vi "Main.vi"(8 "error in":errorcluster, 11 "DataBase in":refnum<class "DataBase.lvclass">) -> (0 "error out":errorcluster, 3 "DataBase out":refnum<class "DataBase.lvclass">)   [LabVIEW 2023, in "DataBase.lvclass"]
doc: "The <b>Queued Message Handler</b> of the Worker that owns this VI."
uses:
  DataBase.lvclass
  C:/Program Files/National Instruments/LabVIEW 2023/vi.lib/addons/_Workers/Library/Classes/Worker/Worker.lvclass
  Items Type.ctl
  rql_Open.ctl
  Initialization Data.ctl
  Response Cases.ctl
  DataBase.lvclass/DataBase.ctl
  rql_Get Last.ctl
  <vilib>/addons/_Workers/Library/Classes/Message Queue/Message Queue.lvclass
  <userlib>/db/db.lvlib
panel:
  out "Items":T1
  in  "Edit Button":bool
  in  "Remove Button":bool
  in  "Add Button":bool
  in  "Listbox":i32(listbox)
  in  "Path Control":path
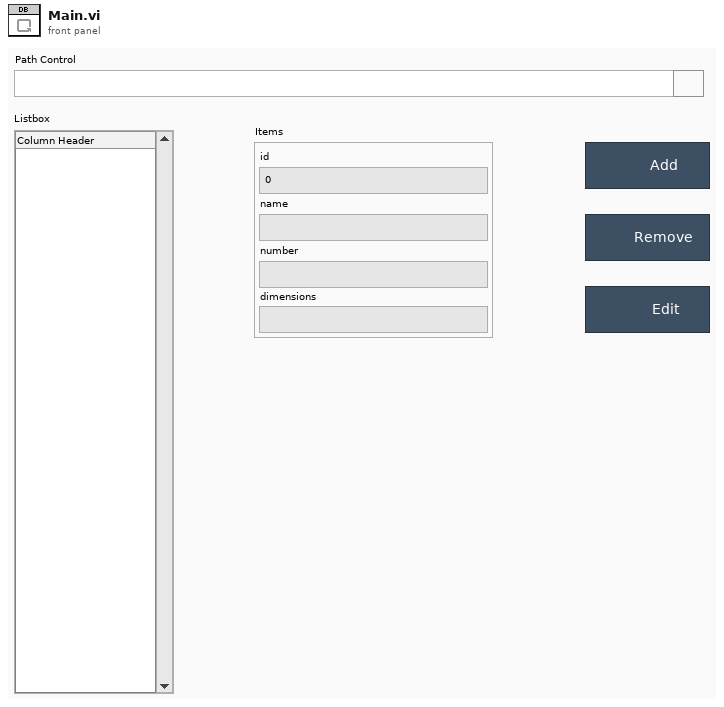
[diagram p1: front panel]
types:
  T1 = typedef "DataBase.lvclass/Items Type.ctl" = cluster{"id":u64, "name":string, "number":string, "dimensions":string}
  T2 = enum32{"Invalid", "Standard", "Closed", "Hidden", "Minimized", "Maximized"}
  T3 = typedef "DataBase.lvclass/Initialization Data.ctl" = cluster{"Response Cases":T4}
  T4 = typedef "DataBase.lvclass/Response Cases.ctl" = cluster{"Placeholder - Can be deleted":string}
  T5 = typedef "DataBase.lvclass/rql_Get Last.ctl" = cluster{"Nums":i32}
  T6 = typedef "DataBase.lvclass/rql_Open.ctl" = cluster{"DB Path":string}
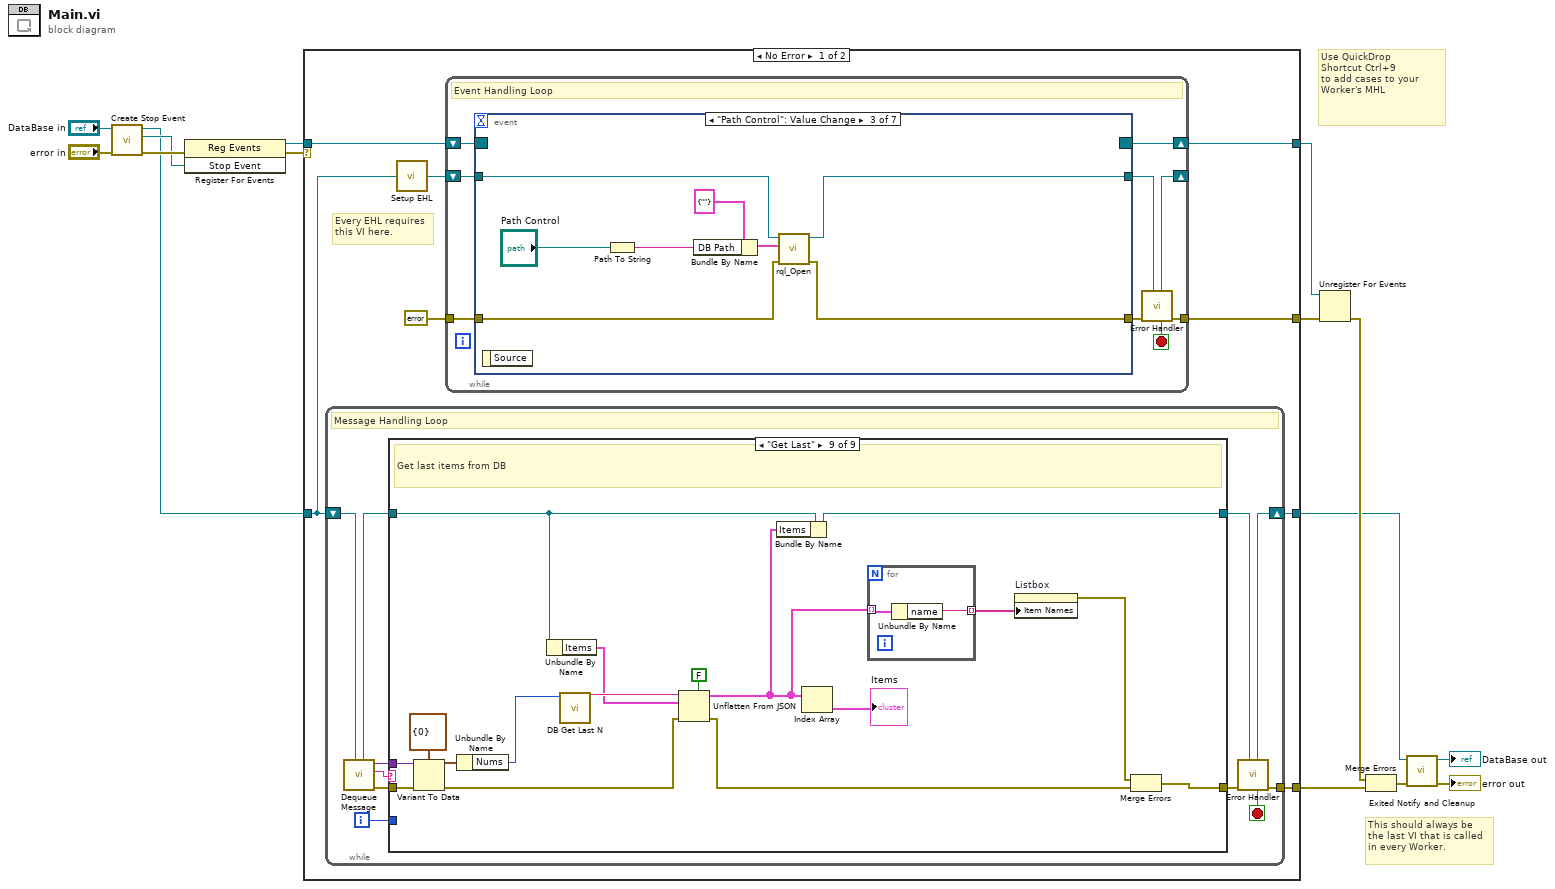
[diagram p0: block diagram]
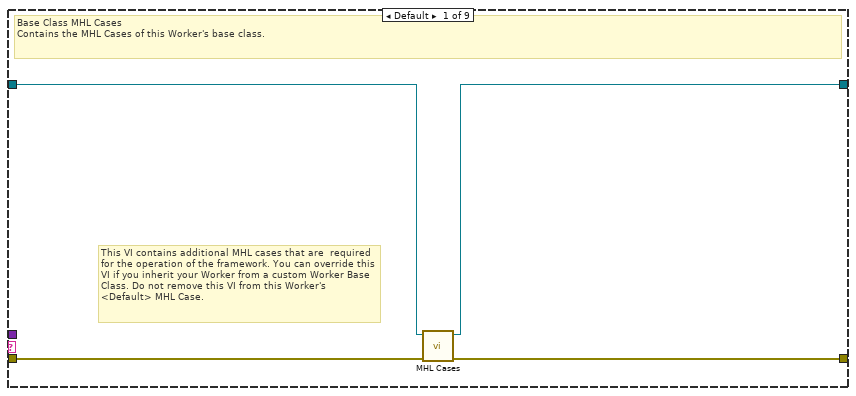
[diagram p2: hidden frame]
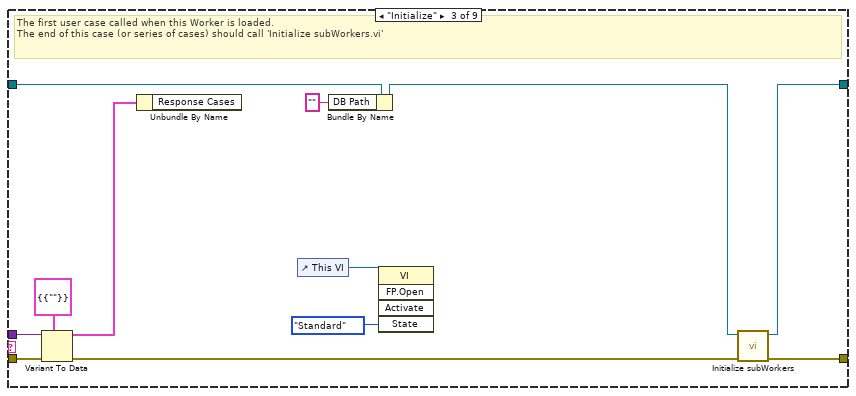
[diagram p4: hidden frame]
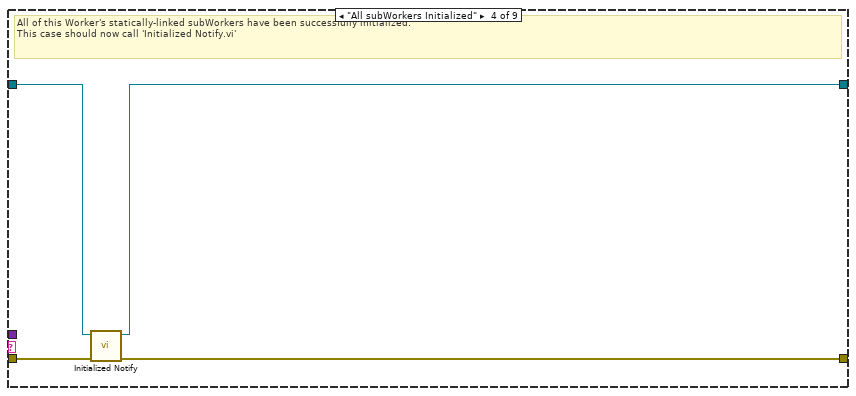
[diagram p5: hidden frame]
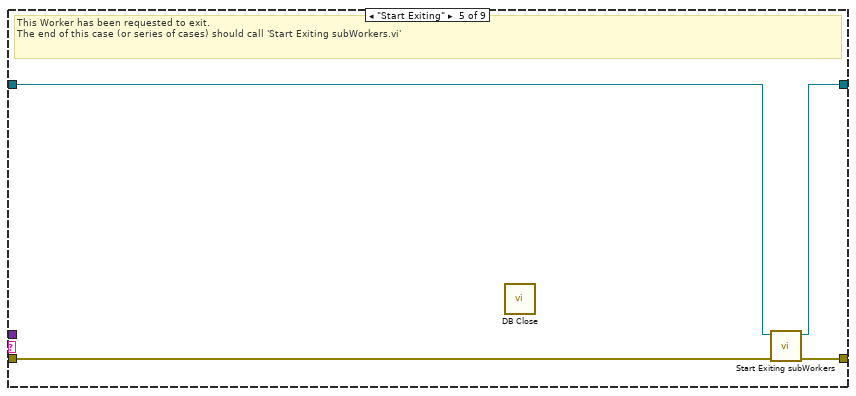
[diagram p6: hidden frame]
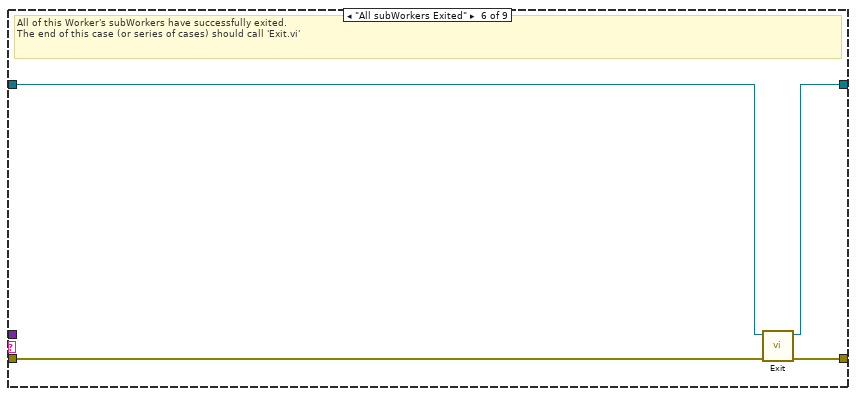
[diagram p7: hidden frame]
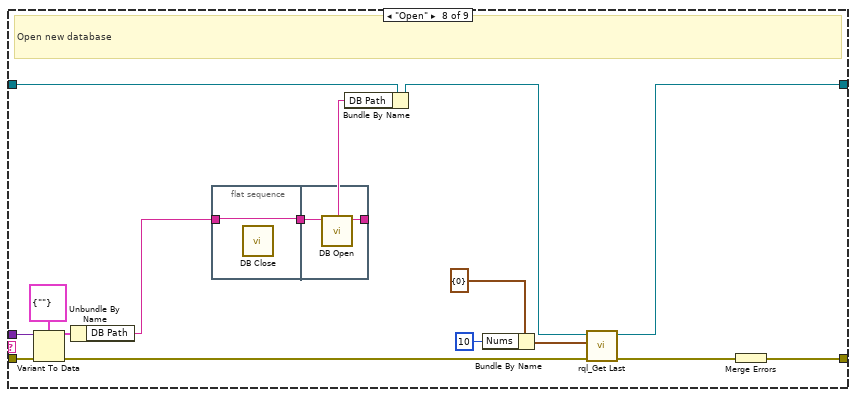
[diagram p9: hidden frame]
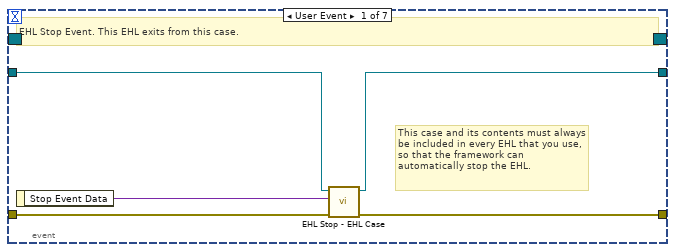
[diagram p10: hidden frame]
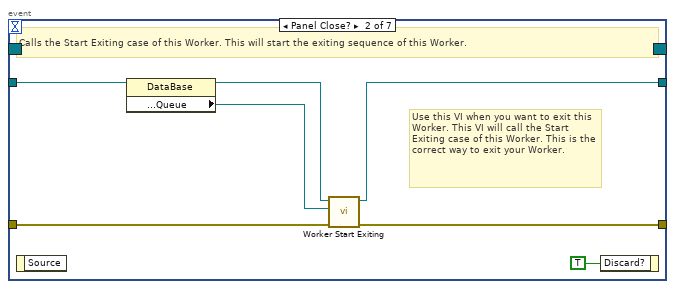
[diagram p11: hidden frame]
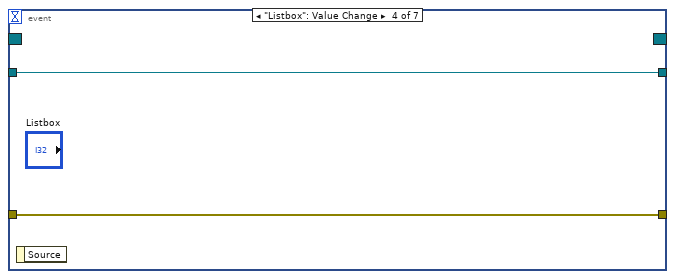
[diagram p12: hidden frame]
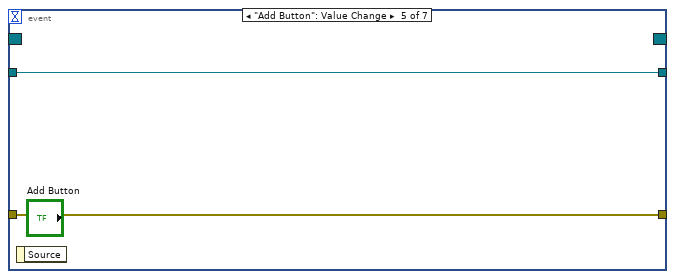
[diagram p13: hidden frame]
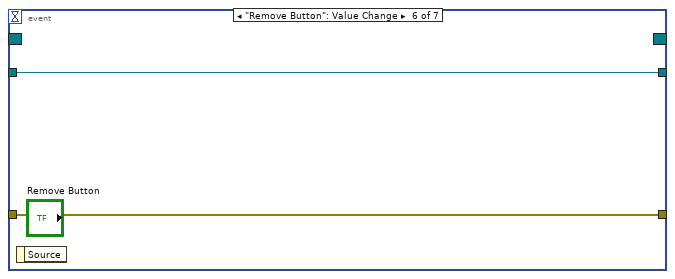
[diagram p14: hidden frame]
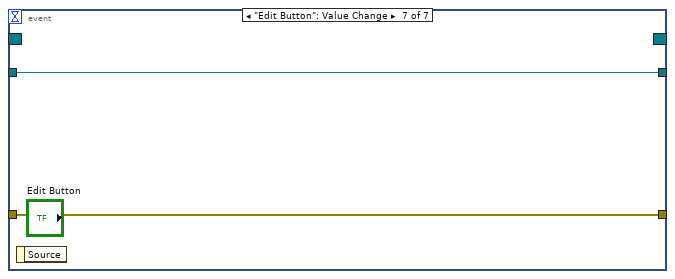
[diagram p15: hidden frame]
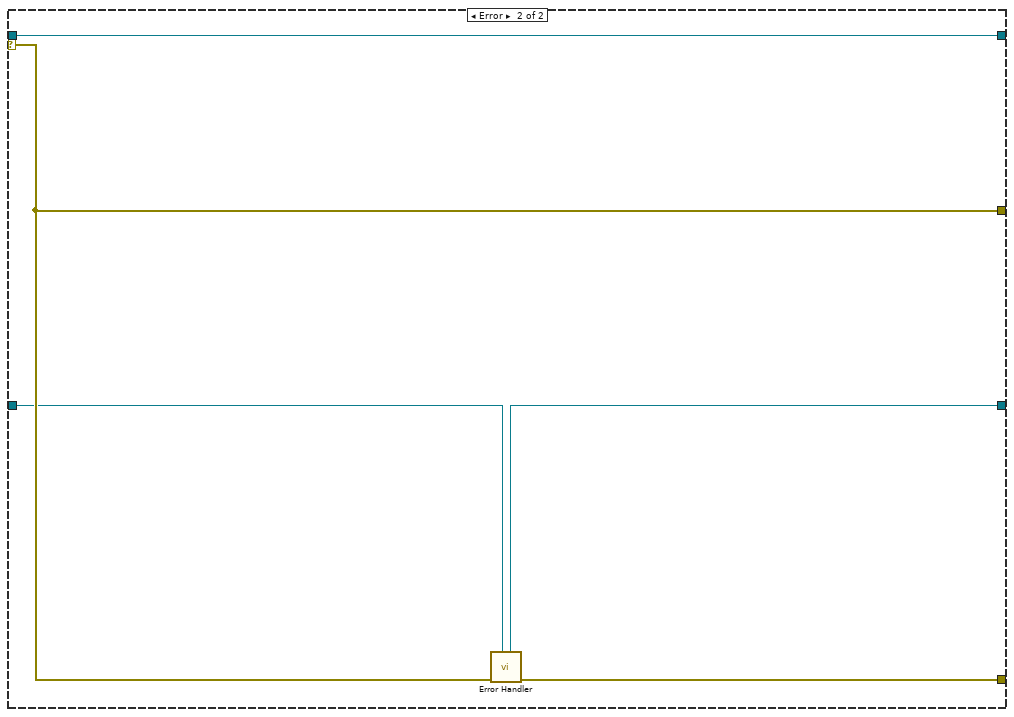
[diagram p16: hidden frame]
diagram:
  # "Use QuickDrop\nShortcut Ctrl+9\nto add cases to your\nWorker's MHL"
  # "This should always be the last VI that is called in every Worker."
  n1 = call-dynamic "Create Stop Event.vi"("error in"="error in", "Worker"="DataBase in") -> ("error out"=w10:errorcluster, "Stop Event"=w7:refnum<user-event>, "Worker out"=w4:refnum<class "DataBase.lvclass">)  [unwired: 7 in]
  n2 = register-events(error in=w10, w7) -> (reference out=w9:refnum<event-registration>, error out=w1:errorcluster)  [unwired: 1 in]
  n3 = case shown="No Error" w1 {
    tunnel: w4 -> [w18 w143]
    tunnel: [w16 w144] -> w8
    tunnel: w9 -> [w23 w145]
    tunnel: [w20 w146] -> w14
    tunnel: [w22 w145] -> w13
    tunnel: [w17 w142] -> w11
    selector: w1 -> [_ w146]
    frame No Error {
      # "Every EHL requires\nthis VI here."
      n4 = while {
        shift-right: [w32] -> w17
        shift-left: w18 -> [w34]
        tunnel: [w33] -> w16
        i -> [w25]
        stop <- w26 stop-if-true
        # "Message Handling Loop"
        n5 = call-dynamic "Dequeue Message.vi"("Worker"=w34) -> ("error out"=w31:errorcluster, "Case out"=w27:string, "Data out"=w24:variant, "Worker out"=w29:refnum<class "DataBase.lvclass">)  [unwired: 6 in, 1 out]
        n6 = case "Worker MHL Case Structure (DO NOT CHANGE LABEL NAME)" shown="\"Get Last\"" w27 {
          tunnel: w31 -> [w38 w39 w50 w54 w57 w64 w66 w81 w102]
          tunnel: [w37 w39 w52 w53 w60 w63 w66 w77 w98] -> w30
          tunnel: w29 -> [w36 w40 w49 w56 w58 w62 w65 w82 w94]
          tunnel: [w35 w40 w51 w55 w59 w61 w65 w73 w89] -> w28
          tunnel: w25 -> [_ _ _ _ _ _ _ _ _]
          tunnel: w24 -> [_ _ w47 _ _ _ _ w79 w100]
          frame Default {
            # "This VI contains additional MHL cases that are  required for the operation of the framework. You can override this VI if you inherit your Worker from a custom Worker Base Class. Do not remove this VI from this Worker's <Default> MHL Case."
            # "Base Class MHL Cases\nContains the MHL Cases of this Worker's base class."
            n7 = call-dynamic "MHL Cases.vi"("error in"=w38, "Worker in"=w36) -> ("error out"=w37:errorcluster, "Worker out"=w35:refnum<class "DataBase.lvclass">)  [unwired: 8 in]
          }
          frame "------------ FRAMEWORK CASES -----------" {
            # "Start of Workers Framework Cases"
          }
          frame "Initialize" {
            # "The first user case called when this Worker is loaded.\nThe end of this case (or series of cases) should call 'Initialize subWorkers.vi'"
            n8 = Variant To Data(error in=w50, type=T3 {"Response Cases"={"Placeholder - Can be deleted"=""}} ("Initialization Data"), Variant=w47) -> (data=w45:T3, error out=w48:errorcluster)
            n9 = Unbundle By Name(w45) -> ()  [unwired: 1 out]
            n10 = control-ref of="This VI"() -> (w41:refnum<vi>)
            n11 = Bundle By Name(cluster=w49, "DB Path"="") -> (w46:refnum<class "DataBase.lvclass">)
            n12 = invoke class="VI" method="FP.Open"(reference=w41, "State"=T2."Standard") -> ()  [unwired: 3 in, 5 out]
            n13 = call-dynamic "Initialize subWorkers.vi"("error in"=w48, "Worker"=w46) -> ("error out"=w52:errorcluster, "dup Worker out"=w51:refnum<class "DataBase.lvclass">)  [unwired: 8 in]
          }
          frame "All subWorkers Initialized" {
            # "All of this Worker's statically-linked subWorkers have been successfully initialized.\nThis case should now call 'Initialized Notify.vi'"
            n14 = call-dynamic "Initialized Notify.vi"("error in"=w54, "Worker"=w56) -> ("error out"=w53:errorcluster, "dup Worker out"=w55:refnum<class "DataBase.lvclass">)  [unwired: 8 in]
          }
          frame "Start Exiting" {
            # "This Worker has been requested to exit. \nThe end of this case (or series of cases) should call 'Start Exiting subWorkers.vi'"
            n15 = call <userlib>:"DB Close.vi"() -> ()  [unwired: 11 in, 1 out]
            n16 = call-dynamic "Start Exiting subWorkers.vi"("error_in"=w57, "Worker"=w58) -> ("error out"=w60:errorcluster, "dup Worker out"=w59:refnum<class "DataBase.lvclass">)  [unwired: 8 in]
          }
          frame "All subWorkers Exited" {
            # "All of this Worker's subWorkers have successfully exited. \nThe end of this case (or series of cases) should call 'Exit.vi'"
            n17 = call-dynamic "Exit.vi"("error_in"=w64, "Worker"=w62) -> ("error out"=w63:errorcluster, "dup Worker out"=w61:refnum<class "DataBase.lvclass">)  [unwired: 8 in]
          }
          frame "------------- LOCAL API CASES -------------" {
            # "Start of Workers Local API Cases"
          }
          frame "Open" {
            # "Open new database"
            n18 = Variant To Data(error in=w81, type=T6 {"DB Path"=""} ("Data"), Variant=w79) -> (data=w78:T6, error out=w75:errorcluster)
            n19 = Unbundle By Name(w78) -> ("DB Path"=w69:string)
            n20 = flat-sequence {
              tunnel: w69 -> [w83]
              tunnel: [w83] -> w67
              tunnel: [w84] -> w68
              tunnel: w67 -> [w85]
              frame #0 {
                n21 = call <userlib>:"DB Close.vi"() -> ()  [unwired: 11 in, 1 out]
              }
              frame #1 {
                n22 = call <userlib>:"DB Open.vi"("path"=w85) -> ("path out"=w84:string)  [unwired: 9 in, 1 out]
              }
            }
            n23 = Bundle By Name(cluster=w82, "DB Path"=w68) -> (w74:refnum<class "DataBase.lvclass">)
            n24 = Bundle By Name(cluster=T5 {"Nums"=0} ("Data in"), "Nums"=10) -> (w71:T5)
            n25 = call "rql_Get Last.vi"("error in"=w75, "Data in"=w71, "DataBase in"=w74) -> ("error out"=w76:errorcluster, "dup DataBase out"=w73:refnum<class "DataBase.lvclass">)  [unwired: 7 in]
            n26 = Merge Errors(w76) -> (w77:errorcluster)
          }
          frame "Get Last" {
            # "Get last items from DB"
            n27 = Variant To Data(error in=w102, type=T5 {"Nums"=0} ("Data"), Variant=w100) -> (data=w99:T5, error out=w93:errorcluster)
            n28 = Unbundle By Name(w99) -> ("Nums"=w97:i32)
            n29 = Unbundle By Name(w94) -> ("Items"=w90:T1[])
            n30 = call <userlib>:"DB Get Last N.vi"("n"=w97) -> ("function return"=w96:string)  [unwired: 10 in]
            n31 = Unflatten From JSON(enable LabVIEW extensions? (T)=FALSE, JSON string=w96, type and defaults=w90, error in (no error)=w93) -> (value=w88:T1[], error out=w92:errorcluster)  [unwired: 3 in]
            n32 = Bundle By Name(cluster=w94, "Items"=w88) -> (w89:refnum<class "DataBase.lvclass">)
            n33 = Index Array(array=w88) -> (element=→"Items":T1)  [unwired: 1 in]
            n34 = for {
              tunnel: w88 -> [w104] mode=indexing
              tunnel: [w103] -> w87 mode=indexing
              n35 = Unbundle By Name(w104) -> ("name"=w103:string)
            }
            n36 = property on="Listbox" class="LstBox (strict)"("Item Names"=w87) -> (error out=w86:errorcluster)  [unwired: 2 in, 1 out]
            n37 = Merge Errors(w86, w92) -> (w98:errorcluster)
          }
        }
        n38 = call-dynamic "Error Handler.vi"("Worker"=w28, "error_in"=w30) -> ("error out"=w33:errorcluster, "Stop Loop"=w26:bool, "Worker out"=w32:refnum<class "DataBase.lvclass">)  [unwired: 7 in]
      }
      n39 = call-dynamic "Setup EHL.vi"("Worker"=w18) -> ("Worker out"=w19:refnum<class "DataBase.lvclass">)  [unwired: 14 in]
      n40 = while "Event Handling Loop" {
        shift-right: [w113] -> w22
        shift-left: w23 -> [w112]
        tunnel: [w108] -> w20
        tunnel: errorcluster {"status"=FALSE, "code"=0, "source"=""} ("error constant") -> [w110]
        shift-right: [w106] -> _
        shift-left: w19 -> [w111]
        stop <- w105 stop-if-true
        # "Event Handling Loop"
        n41 = event shown="[2] \"Path Control\": Value Change" {
          selector: w112 -> [_ _ _ _ _ _ _]
          dyn-events: [_ _ _ _ _ _ _] -> w113
          timeout: _ -> [_ _ _ _ _ _ _]
          tunnel: [w117 w124 w130 w135 w137 w139 w141] -> w109
          tunnel: w110 -> [w118 w123 w131 w135 w137 w139 w141]
          tunnel: w111 -> [w116 w122 w133 w134 w136 w138 w140]
          tunnel: [w115 w121 w132 w134 w136 w138 w140] -> w107
          event User Event {
            # "This case and its contents must always be included in every EHL that you use, so that the framework can automatically stop the EHL."
            # "EHL Stop Event. This EHL exits from this case."
            n42 = event-data() -> ("Stop Event Data"=w114:variant)  [unwired: 1 in]
            n43 = call-dynamic "EHL Stop - EHL Case.vi"("error in"=w118, "Stop Event Data"=w114, "Worker"=w116) -> ("error out"=w117:errorcluster, "Worker out"=w115:refnum<class "DataBase.lvclass">)  [unwired: 7 in]
          }
          event Panel Close? {
            # "Use this VI when you want to exit this Worker. This VI will call the Start Exiting case of this Worker. This is the correct way to exit your Worker."
            # "Calls the Start Exiting case of this Worker. This will start the exiting sequence of this Worker."
            n44 = event-data() -> ()  [unwired: 1 in, 1 out]
            n45 = property class="DataBase"(reference=w122) -> (reference out=w120:refnum<class "DataBase.lvclass">, "Accessors:Read:Public API:Queue"=w119:refnum<class "Message Queue.lvclass">)  [unwired: 1 in, 1 out]
            n46 = call-dynamic "Worker Start Exiting.vi"("error_in"=w123, "Message Queue"=w119, "Worker"=w120) -> ("error out"=w124:errorcluster, "dup Worker out"=w121:refnum<class "DataBase.lvclass">)  [unwired: 7 in]
            n47 = event-data("Discard?"=TRUE) -> ()  [unwired: 1 in, 1 out]
          }
          event "Path Control": Value Change {
            n48 = event-data() -> ()  [unwired: 1 in, 1 out]
            n49 = Path To String(path="Path Control") -> (string=w126:string)
            n50 = Bundle By Name(cluster=T6 {"DB Path"=""} ("Data in"), "DB Path"=w126) -> (w128:T6)
            n51 = call "rql_Open.vi"("error in"=w131, "Data in"=w128, "DataBase in"=w133) -> ("error out"=w130:errorcluster, "dup DataBase out"=w132:refnum<class "DataBase.lvclass">)  [unwired: 7 in]
          }
          event "Listbox": Value Change {
            n52 = event-data() -> ()  [unwired: 1 in, 1 out]
          }
          event "Add Button": Value Change {
            n53 = event-data() -> ()  [unwired: 1 in, 1 out]
          }
          event "Remove Button": Value Change {
            n54 = event-data() -> ()  [unwired: 1 in, 1 out]
          }
          event "Edit Button": Value Change {
            n55 = event-data() -> ()  [unwired: 1 in, 1 out]
          }
        }
        n56 = call-dynamic "Error Handler.vi"("Worker"=w107, "error_in"=w109) -> ("error out"=w108:errorcluster, "Stop Loop"=w105:bool, "Worker out"=w106:refnum<class "DataBase.lvclass">)  [unwired: 7 in]
      }
    }
    frame Error {
      n57 = call-dynamic "Error Handler.vi"("Worker"=w143, "error_in"=w146) -> ("error out"=w144:errorcluster, "Worker out"=w142:refnum<class "DataBase.lvclass">)  [unwired: 7 in, 1 out]
    }
  }
  n58 = Unregister For Events(event registration refnum=w13, error in=w14) -> (error out=w15:errorcluster)
  n59 = Merge Errors(w15, w8) -> (w12:errorcluster)
  n60 = call-dynamic "Exited Notify and Cleanup.vi"("error_in"=w12, "Worker"=w11) -> ("error out"=→"error out":errorcluster, "dup Worker out"=→"DataBase out":refnum<class "DataBase.lvclass">)  [unwired: 8 in]
